vi "PLC.Debug.RandomData.vi"(6 "Delay [s] (1)":dbl=1.0 format="%#_13g", 8 "error in (no error)":errorcluster, 9 "Serial.Component":string, 10 "Serial.Product":string, 11 "Idx":i32) -> (0 "error out":errorcluster)   [LabVIEW 2016]
doc: "Connect to PLC\n\nWabco 2017 All right reserved\nAuthor: maciej.szupienko@wabco-auto.com"
uses:
  Database/Database.Global.vi
  LowLevel/PLC.DataBlock.PLCvalues.ctl
  LowLevel/PLC.DataBlock.PLCcheckstatus.ctl
  Database/ProdaNG/Controls/ProdaNG.TestValue.ctl
panel:
  out "TV":T1[][](array[typedef]) {"minimum" format="%#.3f"; "maximum" format="%#.3f"}
  out "output cluster":T2 {"Values" format="%.3f"}
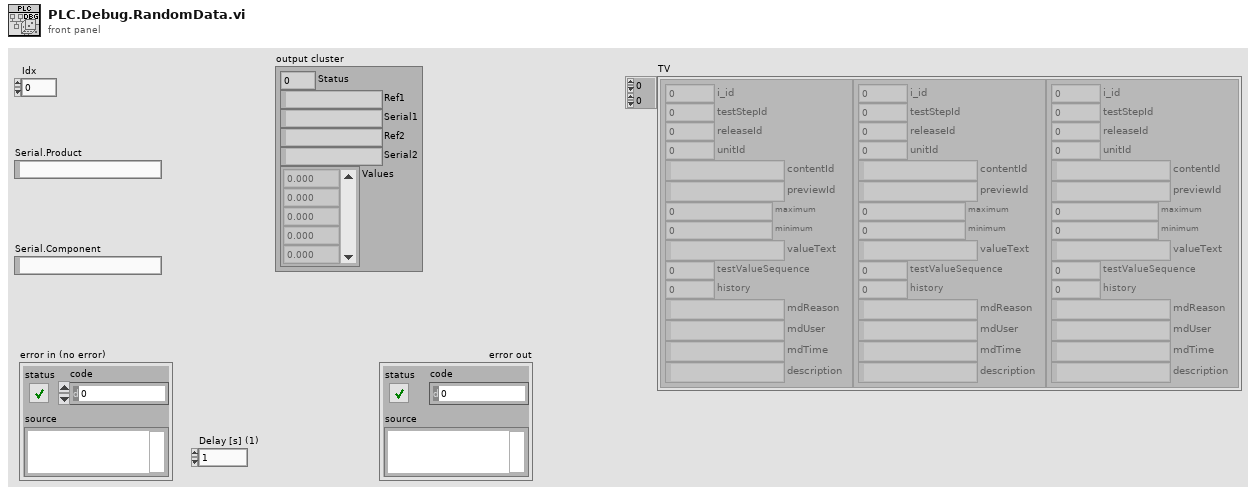
[diagram p1: front panel]
types:
  T1 = typedef "ProdaNG.TestValue.ctl" = cluster{"i_id":i32, "testStepId":i32, "releaseId":i32, "unitId":i32, "contentId":string, "previewId":string, "maximum":dbl, "minimum":dbl, "valueText":string, "testValueSequence":i32, "history":i32, "mdReason":string, "mdUser":string, "mdTime":string, "description":string}
  T2 = typedef "PLC.DataBlock.PLCvalues.ctl" = cluster{"Status":u8, "Ref1":string, "Serial1":string, "Ref2":string, "Serial2":string, "Values":sgl[]}
  T3 = typedef "PLC.DataBlock.PLCcheckstatus.ctl" = cluster{"Ref1":string, "Serial1":string, "Ref2":string, "Serial2":string}
  T4 = typedef "Database.Data.Variant.Sets.ctl" = cluster{"PrevStations":string[], "ThisStations":string[]}
  T5 = typedef "PLC.DataBlock.PCcheckstatus.ctl" = cluster{"Ref":string, "Serial":string, "StatusPrev":i8, "StatusThis":i8, "Repetitions":u8}
  T6 = typedef "Cache.TestSteps.Fglb.ResultData.ctl" = cluster{"File":path, "Ref":string, "Serial":string, "Pr":T7, "PSr":T8, "TSr":cluster{"TSr":T9, "TVr":T10[]}[]}
  T7 = typedef "ProdaNG.ProcessResult.ctl" = cluster{"c_id":string, "productId":string, "processId":i32, "statusId":i32, "startTime":string, "endTime":string}
  T8 = typedef "ProdaNG.ProcessStepResult.ctl" = cluster{"c_id":string, "processResultId":string, "processStepId":i32, "statusId":i32, "operatorId":i32, "startTime":string, "endTime":string}
  T9 = typedef "ProdaNG.TestStepResult.ctl" = cluster{"c_id":string, "processStepResultId":string, "testStepId":i32, "statusId":i32}
  T10 = typedef "ProdaNG.TestValueResult.ctl" = cluster{"c_id":string, "testStepResultId":string, "testValueId":i32, "result":dbl, "statusId":i32, "contentId":string}
  T11 = typedef "Cache.TestSteps.Fglb.TestData.ctl" = cluster{"Ref":string, "Desc":string, "P":T12, "PS":T13, "PP":T14[], "TS":cluster{"TS":T15, "TV":T1[], "TP":T16[]}[], "Units":T17[]}
  T12 = typedef "ProdaNG.Process.ctl" = cluster{"i_id":i32, "productionLineId":i32, "releaseId":i32, "contentId":string, "previewId":string, "mdReason":string, "mdUser":string, "mdTime":string, "description":string}
  T13 = typedef "ProdaNG.ProcessStep.ctl" = cluster{"i_id":i32, "processId":i32, "systemId":i32, "releaseId":i32, "processSequence":i32, "limitYellow":dbl, "limitRed":dbl, "mdReason":string, "mdUser":string, "mdTime":string, "filename":string, "transfer":string, "description":string}
  T14 = typedef "ProdaNG.ProcessStepParam.ctl" = cluster{"i_id":i32, "processStepId":i32, "unitId":i32, "contentId":string, "previewId":string, "value":dbl, "valueText":string, "paramSequence":i32, "history":i32, "mdReason":string, "mdUser":string, "mdTime":string, "description":string}
  T15 = typedef "ProdaNG.TestStep.ctl" = cluster{"i_id":i32, "processStepId":i32, "testSequence":i32, "testOrder":i32, "mdReason":string, "mdUser":string, "mdTime":string, "description":string}
  T16 = typedef "ProdaNG.TestStepParam.ctl" = cluster{"i_id":i32, "testStepId":i32, "unitId":i32, "contentId":string, "previewId":string, "value":dbl, "valueText":string, "paramSequence":i32, "history":i32, "mdReason":string, "mdUser":string, "mdTime":string, "description":string}
  T17 = typedef "ProdaNG.Unit.ctl" = cluster{"i_id":i32, "name":string, "mdReason":string, "mdUser":string, "mdTime":string, "description":string}
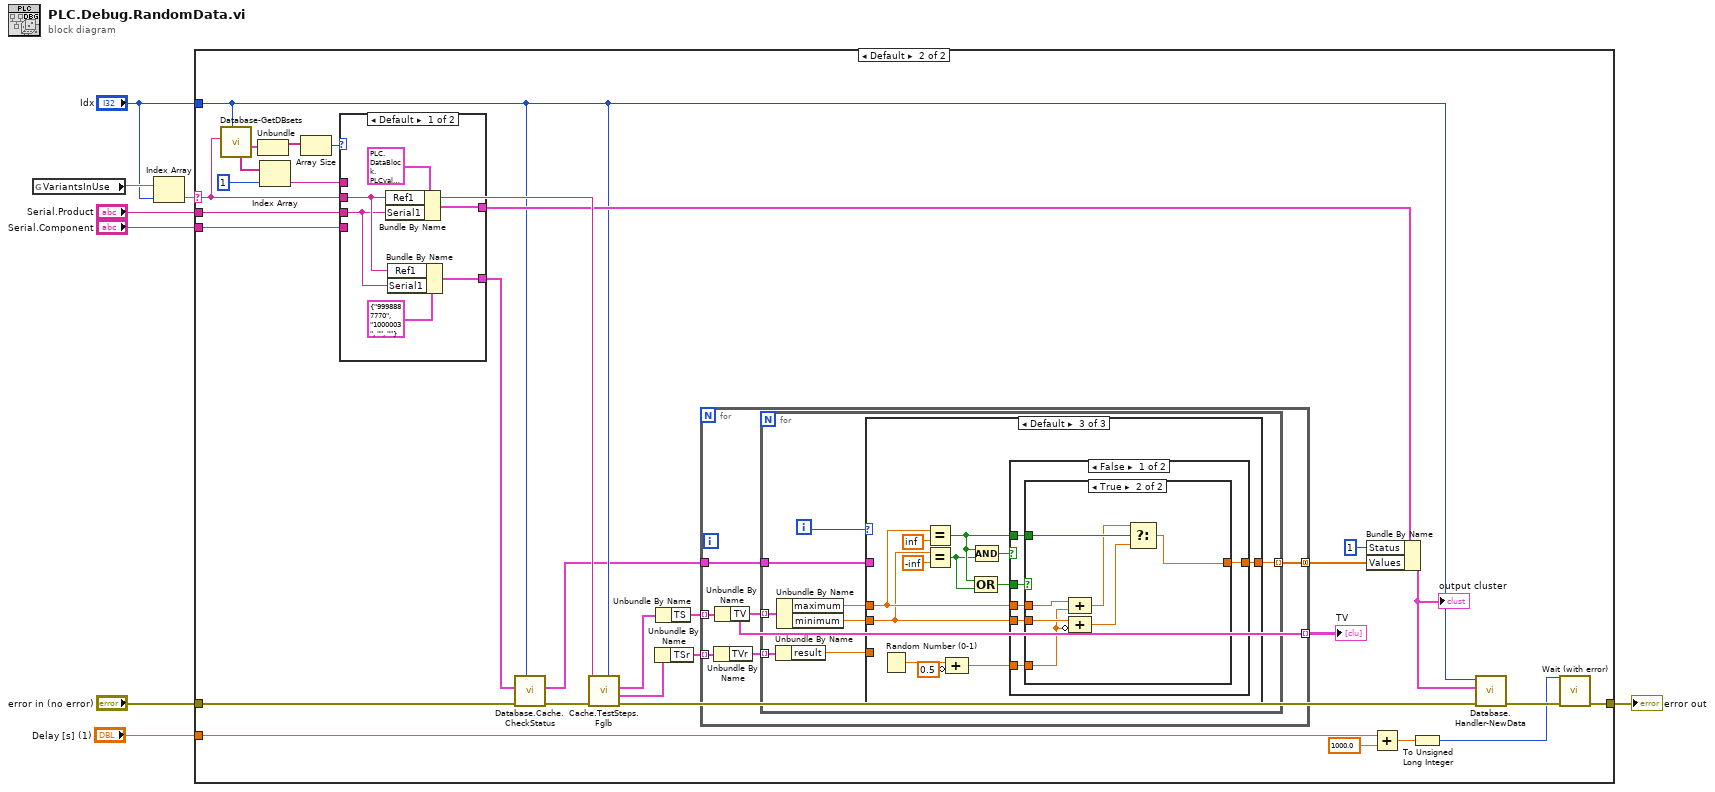
[diagram p0: block diagram]
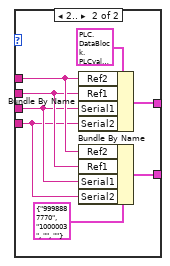
[diagram p3: hidden frame]
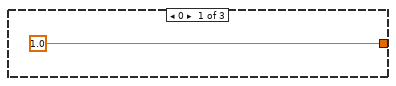
[diagram p4: hidden frame]
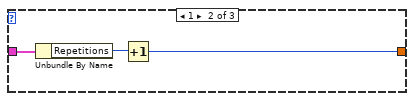
[diagram p5: hidden frame]
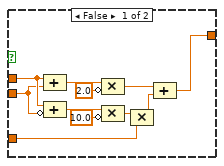
[diagram p6: hidden frame]
diagram:
  n1 = global read "Database.Global.vi" "VariantsInUse"() -> (w6)
  n2 = Index Array(array=w6, index="Idx") -> (element=w4)
  n3 = case shown="Default" w4 {
    selector: w4 -> [_ w36]
    tunnel: [w9 w23] -> w8
    tunnel: "error in (no error)" -> [w9 w13]
    tunnel: "Idx" -> [_ w14]
    tunnel: "Serial.Product" -> [_ w29]
    tunnel: "Serial.Component" -> [_ w28]
    tunnel: "Delay [s] (1)" -> [_ w22]
    frame "" {
    }
    frame Default {
      n4 = call "Database-GetDBsets.vi"("Idx"=w14, "Variant"=w36) -> ("Variant Sets"=w35:T4, "PrevVariantsInUse"=w33:string[])  [unwired: 5 in, 3 out]
      n5 = Unbundle(w35) -> ("PrevStations"=w34:string[])  [unwired: 1 out]
      n6 = Index Array(array=w33, index=1) -> (element=w31:string)
      n7 = Array Size(array=w34) -> (size(s)=w30:i32)
      n8 = case shown="Default" w30 {
        tunnel: w36 -> [w43 w50]
        tunnel: [w44 w52] -> w15
        tunnel: w31 -> [_ w51]
        tunnel: w29 -> [w42 w49]
        tunnel: w28 -> [_ w48]
        tunnel: [w41 w46] -> w11
        frame Default {
          n9 = Bundle By Name(cluster=T2 {"Status"=0, "Ref1"="9998887770", "Serial1"="12345679", "Ref2"="", "Serial2"="", "Values"=[1.0, 2.0, 1.0, 1.0, 1.0, 4.0, 5.0, 1.0]} ("Data"), "Ref1"=w43, "Serial1"=w42) -> (w44:T2)
          n10 = Bundle By Name(cluster=T3 {"Ref1"="9998887770", "Serial1"="1000003", "Ref2"="", "Serial2"=""} ("Data in"), "Ref1"=w43, "Serial1"=w42) -> (w41:T3)
        }
        frame 2.. {
          n11 = Bundle By Name(cluster=T2 {"Status"=0, "Ref1"="9998887770", "Serial1"="12345679", "Ref2"="", "Serial2"="", "Values"=[1.0, 2.0, 1.0, 1.0, 1.0, 4.0, 5.0, 1.0]} ("Data"), "Ref2"=w51, "Ref1"=w50, "Serial1"=w49, "Serial2"=w48) -> (w52:T2)
          n12 = Bundle By Name(cluster=T3 {"Ref1"="9998887770", "Serial1"="1000003", "Ref2"="", "Serial2"=""} ("Data in"), "Ref2"=w51, "Ref1"=w50, "Serial1"=w49, "Serial2"=w48) -> (w46:T3)
        }
      }
      n13 = call "Database.Cache.CheckStatus.vi"("Idx"=w14, "error in"=w13, "Data in"=w11) -> ("error out"=w12:errorcluster, "Data out"=w10:T5)  [unwired: 7 in]
      n14 = call "Cache.TestSteps.Fglb.vi"("SystemIdx"=w14, "error in (no error)"=w12, "Variant"=w36) -> ("error out"=w37:errorcluster, "Result out"=w39:T6, "Test out"=w17:T11)  [unwired: 5 in, 1 out]
      n15 = Unbundle By Name(w39) -> ("TSr"=w38:cluster{"TSr":T9, "TVr":T10[]}[])
      n16 = Unbundle By Name(w17) -> ("TS"=w18:cluster{"TS":T15, "TV":T1[], "TP":T16[]}[])
      n17 = for {
        tunnel: w38 -> [w59] mode=indexing
        tunnel: [w57] -> w27 mode=concatenating
        tunnel: w18 -> [w56] mode=indexing
        tunnel: [w55] -> w16 mode=indexing
        tunnel: w10 -> [w54]
        n18 = Unbundle By Name(w59) -> ("TVr"=w58:T10[])
        n19 = Unbundle By Name(w56) -> ("TV"=w55:T1[])
        n20 = for {
          tunnel: w58 -> [w67] mode=indexing
          tunnel: [w66] -> w57 mode=indexing
          tunnel: w55 -> [w62] mode=indexing
          tunnel: w54 -> [w60]
          i -> [w65]
          n21 = Unbundle By Name(w67) -> ("result"=w64:dbl)
          n22 = Unbundle By Name(w62) -> ("maximum"=w63:dbl, "minimum"=w61:dbl)
          n23 = case shown="Default" w65 {
            tunnel: [1.0 w71 w74] -> w66
            tunnel: w64 -> [_ _ _]
            tunnel: w63 -> [_ _ w79]
            tunnel: w61 -> [_ _ w78]
            tunnel: w60 -> [_ w70 _]
            frame 0 {
            }
            frame 1 {
              n24 = Unbundle By Name(w70) -> ("Repetitions"=w69:u8)
              n25 = Increment(x=w69) -> (x+1=w71:u8)
            }
            frame Default {
              n26 = Random Number (0-1)() -> (number: 0 to 1=w76:dbl)
              n27 = Equal?(x=w79, y=inf) -> (x = y?=w73:bool)
              n28 = Equal?(x=w78, y=-inf) -> (x = y?=w72:bool)
              n29 = Compound Arithmetic op=ADD(w76, invert 0.5 ("value")) -> (w75:dbl)
              n30 = Compound Arithmetic op=OR(w73, w72) -> (w80:bool)
              n31 = Compound Arithmetic op=AND(w73, w72) -> (w81:bool)
              n32 = case shown="False" w81 {
                tunnel: w73 -> [w84 _]
                tunnel: w80 -> [w89 _]
                tunnel: w79 -> [w88 _]
                tunnel: w78 -> [w87 _]
                tunnel: w75 -> [w86 w108]
                tunnel: [w85 w108] -> w74
                frame False {
                  n33 = case shown="True" w89 {
                    tunnel: w88 -> [w93 w106]
                    tunnel: w87 -> [w92 w105]
                    tunnel: w86 -> [w91 w103]
                    tunnel: [w90 w101] -> w85
                    tunnel: w84 -> [_ w107]
                    frame False {
                      n34 = Compound Arithmetic op=ADD(w93, w92) -> (w97:dbl)
                      n35 = Compound Arithmetic op=ADD(w93, invert w92) -> (w98:dbl)
                      n36 = Compound Arithmetic op=MULTIPLY(w97, invert 2.0 ("value")) -> (w95:dbl)
                      n37 = Compound Arithmetic op=MULTIPLY(w98, invert 10.0 ("value")) -> (w96:dbl)
                      n38 = Compound Arithmetic op=MULTIPLY(w96, w91) -> (w94:dbl)
                      n39 = Compound Arithmetic op=ADD(w95, w94) -> (w90:dbl)
                    }
                    frame True {
                      n40 = Compound Arithmetic op=ADD(w106, w103) -> (w104:dbl)
                      n41 = Compound Arithmetic op=ADD(w105, invert w103) -> (w102:dbl)
                      n42 = Select(t=w104, s=w107, f=w102) -> (s? t:f=w101:dbl)
                    }
                  }
                }
                frame True {
                }
              }
            }
          }
        }
      }
      "TV" <- w16
      n43 = Bundle By Name(cluster=w15, "Status"=u8 1, "Values"=w27) -> (w26:T2)
      "output cluster" <- w26
      n44 = Add(x=w22, y=1000.0) -> (x+y=w20:dbl)
      n45 = To Unsigned Long Integer(number=w20) -> (unsigned 32bit integer=w19:u32)
      n46 = call "Database.Handler-NewData.vi"("error in"=w37, "Data"=w26, "Idx"=w14) -> ("error out"=w24:errorcluster)  [unwired: 7 in, 1 out]
      n47 = call "Wait (with error).vi"("error in (no error)"=w24, "milliseconds to wait"=w19) -> ("error out"=w23:errorcluster)  [unwired: 8 in, 1 out]
    }
  }
  "error out" <- w8
